vi "TwGetSpecXaxisFromH5.vi"(4 "writeIndex":i32, 5 "error in (no error)":errorcluster, 6 "maxMass":dbl, 7 "axisType":i32, 8 "specAxis in":dbl[](array[numeric]), 9 "filename":string) -> (1 "unitLabel":string, 2 "specAxis out":dbl[](array[numeric]), 3 "error out":errorcluster)   [LabVIEW 2009]
uses:
  TwH5Dll.dll
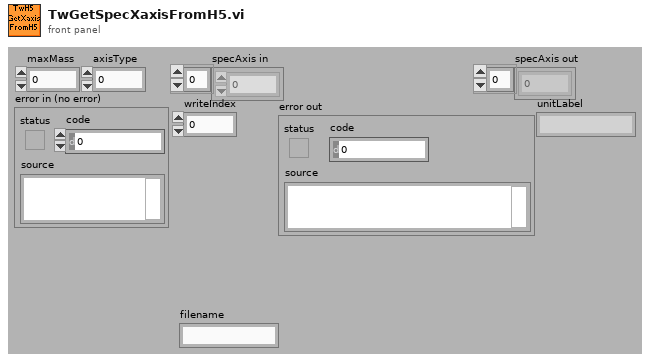
[diagram p1: front panel]
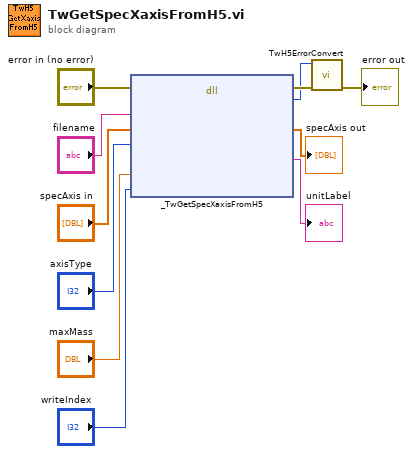
[diagram p0: block diagram]
diagram:
  n1 = dll-call lib="C:/src/85_TofDaq_current/DllWrappers/LabView/TwH5Dll/TwH5Dll.dll" fn="_TwGetSpecXaxisFromH5"(error in="error in (no error)", "filename"="filename", "specAxis"="specAxis in", "axisType"="axisType", "maxMass"="maxMass", "writeIndex"="writeIndex") -> (error out=w10:errorcluster, "TwRetVal"=w9:i32, "specAxis"=→"specAxis out":dbl[], "unitLabel"=→"unitLabel":string)  [unwired: 6 in, 2 out]
  n2 = call "TwH5ErrorConvert.vi"("error in (no error)"=w10, "error code"=w9) -> ("error out"=→"error out":errorcluster)  [unwired: 9 out]
